vi "modelNames.vi"(6 "modelNames (in)":string[](array[string]), 10 "d":i32, 11 "n":i32) -> (3 "modelNames (out)":string[](array[string]))   [LabVIEW 2014]
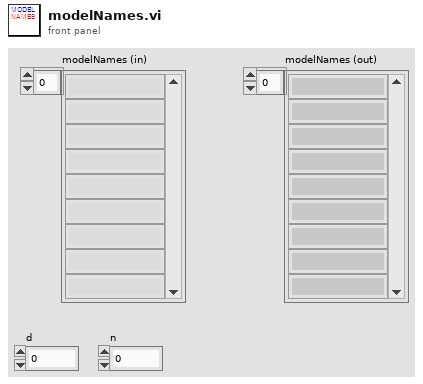
[diagram p1: front panel]
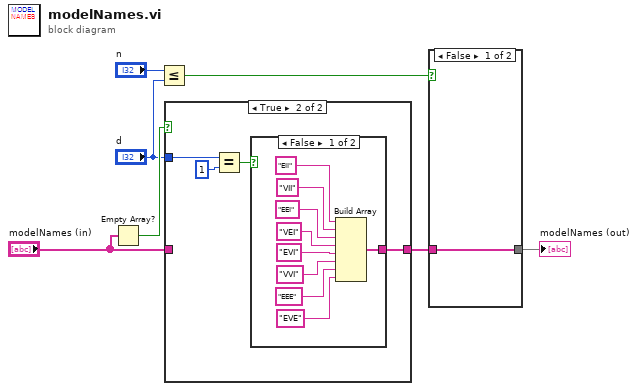
[diagram p0: block diagram]
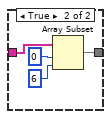
[diagram p2: hidden frame]
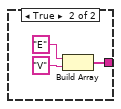
[diagram p4: hidden frame]
diagram:
  n1 = Empty Array?(array="modelNames (in)") -> (empty?=w7:bool)
  n2 = Less Or Equal?(x="n", y="d") -> (x <= y?=w3:bool)
  n3 = case shown="True" w7 {
    tunnel: "d" -> [_ w12]
    tunnel: "modelNames (in)" -> [w8 _]
    tunnel: [w8 w9] -> w2
    frame False {
    }
    frame True {
      n4 = Equal?(x=w12, y=1) -> (x = y?=w10:bool)
      n5 = case shown="False" w10 {
        tunnel: [w21 w22] -> w9
        frame False {
          n6 = Build Array("EII", "VII", "EEI", "VEI", "EVI", "VVI", "EEE", "EVE") -> (w21:string[])
        }
        frame True {
          n7 = Build Array("E", "V") -> (w22:string[])
        }
      }
    }
  }
  n8 = case shown="False" w3 {
    tunnel: w2 -> [w25 w29]
    tunnel: [w25 w26] -> w1
    frame False {
    }
    frame True {
      n9 = Array Subset(array=w29, index=0, length=6) -> (w26:string[])
    }
  }
  "modelNames (out)" <- w1
